vi "Read ASCII or Unicode.vi"(8 "error in (no error)":errorcluster, 11 "Font Class in":refnum<class "Font Class.lvclass">) -> (0 "error out":errorcluster, 1 "ASCII or Unicode":T1, 2 "Type and encoding":T4, 3 "Font Class out":refnum<class "Font Class.lvclass">)   [LabVIEW 2019, in "Font Class.lvclass"]
uses:
  <userlib>/Exaprom PDF/LV Class/Fonts Class/Font Class.lvclass
  <userlib>/Exaprom PDF/Controls/Text Controls/Unicode/Character type with Select.ctl
  <userlib>/Exaprom PDF/Controls/Text Controls/Unicode/Writing direction with Select.ctl
  <userlib>/Exaprom PDF/Controls/Text Controls/Unicode/ASCII or Unicode with Select.ctl
  <userlib>/Exaprom PDF/Controls/Text Controls/Unicode/Type and run direction.ctl
  <userlib>/Exaprom PDF/Controls/Font Controls/Type and encoding.ctl
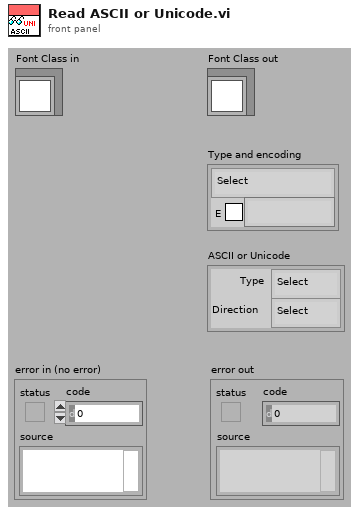
[diagram p1: front panel]
types:
  T1 = typedef "ASCII or Unicode with Select.ctl" = cluster{"Type":T2, "Direction":T3}
  T2 = typedef "Character type with Select.ctl" = enum16{"Select", "ASCII", "Unicode"}
  T3 = typedef "Writing direction with Select.ctl" = enum16{"Select", "Default", "NO BIDI", "LTR", "RTL"}
  T4 = typedef "Type and encoding.ctl" = cluster{"Type&direction":T5, "Embedded":bool, "Encoding":string}
  T5 = typedef "Type and run direction.ctl" = enum16{"Select", "ASCII", "UTF-16", "UTF-16 (default)", "UTF-16 (LTR)", "UTF-16 (RTL)"}
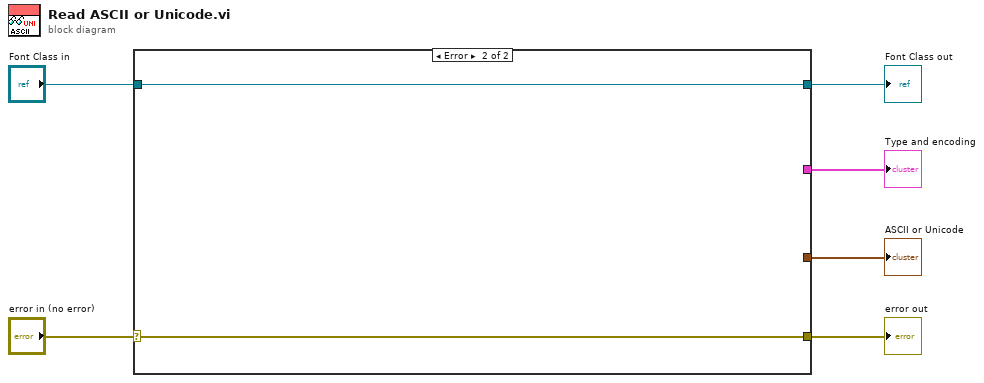
[diagram p0: block diagram]
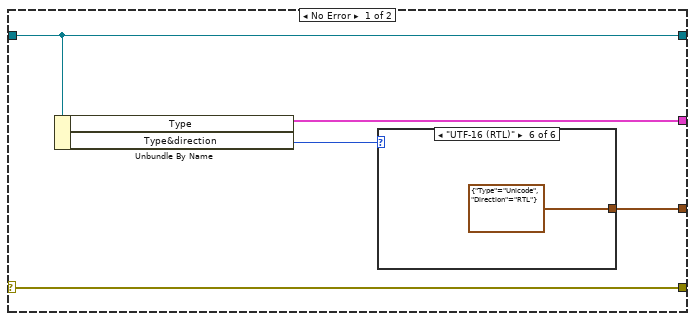
[diagram p2: hidden frame]
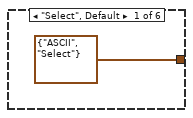
[diagram p3: hidden frame]
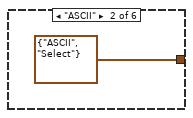
[diagram p4: hidden frame]
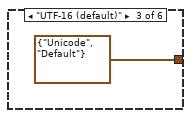
[diagram p5: hidden frame]
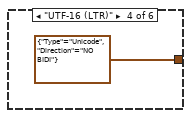
[diagram p6: hidden frame]
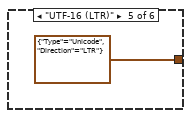
[diagram p7: hidden frame]
diagram:
  n1 = case shown="Error" "error in (no error)" {
    selector: "error in (no error)" -> [w11 w18]
    tunnel: [w11 w18] -> w5
    tunnel: [w10 w19] -> w3
    tunnel: "Font Class in" -> [w10 w19]
    tunnel: [w9 _] -> w2
    tunnel: [w7 _] -> w1
    frame No Error {
      n2 = Unbundle By Name(w10) -> ("Type"=w9:T4, "Type&direction"=w8:T5)
      n3 = case shown="\"UTF-16 (RTL)\"" w8 {
        tunnel: [T1 {"Type"=enum."ASCII", "Direction"=enum."Select"} ("ASCII or Unicode") T1 {"Type"=enum."ASCII", "Direction"=enum."Select"} ("ASCII or Unicode") T1 {"Type"=enum."Unicode", "Direction"=enum."Default"} ("ASCII or Unicode") T1 {"Type"=enum."Unicode", "Direction"=enum."NO BIDI"} ("ASCII or Unicode") T1 {"Type"=enum."Unicode", "Direction"=enum."LTR"} ("ASCII or Unicode") T1 {"Type"=enum."Unicode", "Direction"=enum."RTL"} ("ASCII or Unicode")] -> w7
        frame "Select", Default {
        }
        frame "ASCII" {
        }
        frame "UTF-16 (default)" {
        }
        frame "UTF-16 (LTR)" {
        }
        frame "UTF-16 (LTR)" {
        }
        frame "UTF-16 (RTL)" {
        }
      }
    }
    frame Error {
    }
  }
  "error out" <- w5
  "Font Class out" <- w3
  "Type and encoding" <- w2
  "ASCII or Unicode" <- w1
